vi "FTW-Test-Socket-Stress-PublisherShutdown.vi"() -> (0 "Test Result":errorcluster)   [LabVIEW 2015]
panel:
  out "Endpoints":string[](array[string])
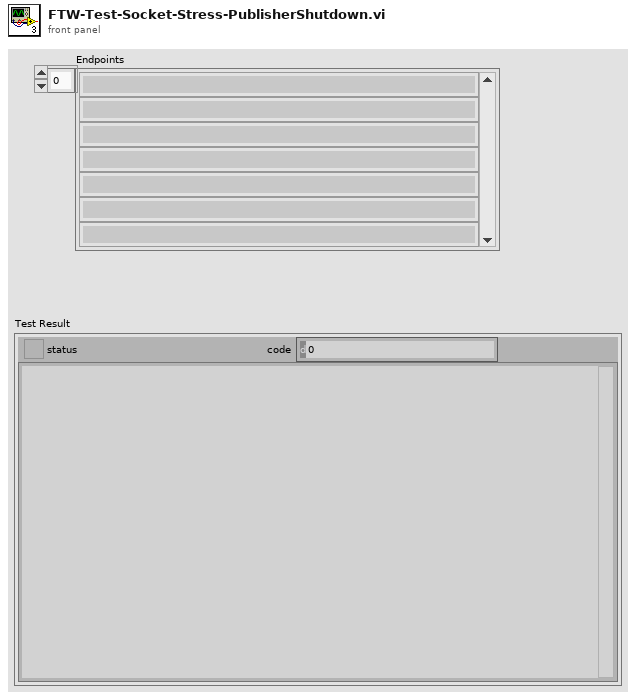
[diagram p1: front panel]
types:
  T1 = typedef "FTW-Type-Socket-Publisher.ctl" = refnum<data-value>
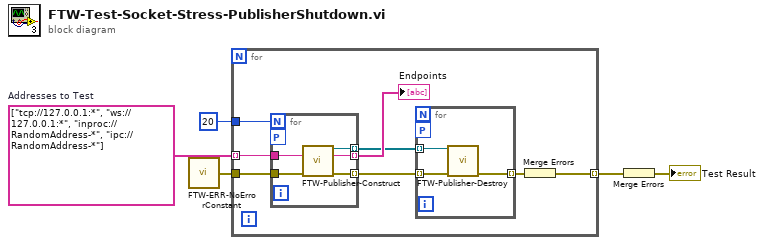
[diagram p0: block diagram]
diagram:
  w5 = string[] ["tcp://127.0.0.1:*", "ws://127.0.0.1:*", "inproc://RandomAddress-*", "ipc://RandomAddress-*"]  # Addresses to Test
  n1 = call "FTW-ERR-NoErrorConstant.vi"() -> ("no error"=w1:errorcluster)
  n2 = for {
    tunnel: [w7] -> w3 mode=indexing
    tunnel: w5 -> [w9] mode=indexing
    tunnel: 20 -> [w8]
    tunnel: w1 -> [w6]
    n3 = for {
      N: w8 -> [_]
      tunnel: [w21] -> w10 mode=indexing
      tunnel: [w20] -> w11 mode=indexing
      tunnel: [w19] -> w13 mode=indexing
      tunnel: w9 -> [w18]
      workers-P: _ -> [_]
      tunnel: w6 -> [w17]
      n4 = call "FTW-Publisher-Construct.vi"("Instance Inbox Address"=w18, "error in"=w17) -> ("Publisher"=w21:T1, "Resolved Inbox Address"=w20:string, "error out"=w19:errorcluster)  [unwired: 11 in]
    }
    "Endpoints" <- w11
    n5 = for {
      tunnel: w10 -> [w16] mode=indexing
      tunnel: w13 -> [w15] mode=indexing
      tunnel: [w14] -> w12 mode=indexing
      workers-P: _ -> [_]
      n6 = call "FTW-Publisher-Destroy.vi"("Publisher"=w16, "error in"=w15) -> ("error out"=w14:errorcluster)  [unwired: 13 in]
    }
    n7 = Merge Errors(w12) -> (w7:errorcluster)
  }
  n8 = Merge Errors(w3) -> (→"Test Result":errorcluster)
